vi "ModeTmeoutSelector.vi"(11 "timeout/wait period (ms)":i32) -> (3 "timeout to use":i32)   [LabVIEW 2017, in "Subsystem.lvclass"]
uses:
  Subsystem.lvclass
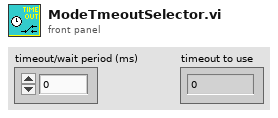
[diagram p1: front panel]
types:
  T1 = typedef "RobotSubsystem.lvclass/RunMode.ctl" = enum16{"Auto", "Teleop", "Disabled"}
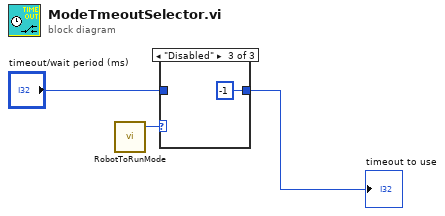
[diagram p0: block diagram]
diagram:
  n1 = call "RobotToRunMode.vi"() -> ("Mode Out"=w3:T1)  [unwired: 11 in]
  n2 = case shown="\"Disabled\"" w3 {
    tunnel: "timeout/wait period (ms)" -> [w4 w5 _]
    tunnel: [w4 w5 -1 ("timeout in ms (-1)")] -> w1
    frame "Auto", Default {
    }
    frame "Teleop" {
    }
    frame "Disabled" {
    }
  }
  "timeout to use" <- w1
